vi "ReadViRef.vi"(8 "error in (no error)":errorcluster caption="错误输入（无错误）", 11 "User Worker 输入":refnum<class "User Worker.lvclass">) -> (0 "error out":errorcluster caption="错误输出", 2 "VI":refnum<vi>, 3 "User Worker 输出":refnum<class "User Worker.lvclass">)   [LabVIEW 2018, in "User Worker.lvclass"]
uses:
  User Worker.lvclass
  User Worker.lvclass/User Worker.ctl
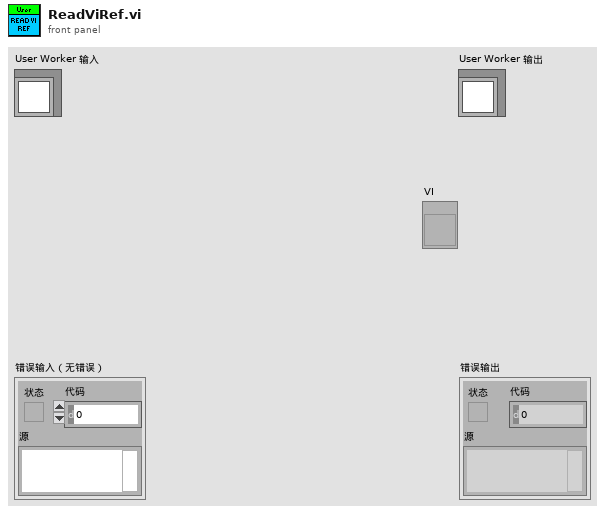
[diagram p1: front panel]
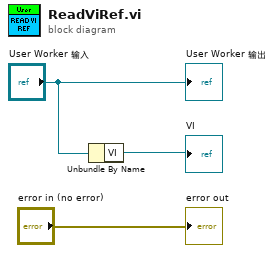
[diagram p0: block diagram]
diagram:
  n1 = Unbundle By Name("User Worker 输入") -> ("VI"=→"VI":refnum<vi>)
  "error out" <- "error in (no error)"
  "User Worker 输出" <- "User Worker 输入"
